vi "Project.vi"(7 "Config in":refnum<class "TAF Proj Config.lvclass">, 8 "error in":errorcluster, 11 "Project":refnum<vi>) -> (0 "error out":errorcluster, 3 "Targets":T1[](array[typedef]))   [LabVIEW 2021, in "TAF Proj Document Type.lvlib" / "Project Parser.lvlib"]
uses:
  <vilib>/Wovalab/AntiDoc/Document Type/Add-ons/LabVIEW TAF Project/Project Parser/Project Parser.lvlib
  <vilib>/Wovalab/AntiDoc/Document Type/Add-ons/LabVIEW TAF Project/TAF Proj Config/TAF Proj Config.lvclass
  <vilib>/Wovalab/AntiDoc/Document Type/Add-ons/LabVIEW TAF Project/Project Parser/Target--cluster.ctl
  <vilib>/Wovalab/AntiDoc/Document Type/Add-ons/LabVIEW TAF Project/Custom Errors/Custom Errors.lvclass
  <vilib>/Wovalab/AntiDoc/Document Type/Add-ons/LabVIEW TAF Project/Classes Overview/Classes Overview.lvclass
  <vilib>/Wovalab/AntiDoc/Document Type/Add-ons/LabVIEW TAF Project/Dqmh Modules Overview/Dqmh Modules Overview.lvclass
  <vilib>/Wovalab/AntiDoc/Document Type/Add-ons/LabVIEW TAF Project/FrontPanelGUI/FrontPanelGUI.lvclass
  <vilib>/Wovalab/AntiDoc/Document Type/Add-ons/LabVIEW TAF Project/Project Parser/Blocs--cluster.ctl
  <vilib>/Wovalab/AntiDoc/Document Type/Add-ons/LabVIEW TAF Project/Dqmh Module/Dqmh Module.lvclass
  <vilib>/Wovalab/AntiDoc/Document Type/Add-ons/LabVIEW TAF Project/Class/Class.lvclass
  <vilib>/Wovalab/AntiDoc/Document Type/Add-ons/LabVIEW TAF Project/Lib/Lib.lvclass
  <vilib>/Wovalab/AntiDoc/Document Type/Add-ons/LabVIEW TAF Project/TAFConfiguration/TAFConfiguration.lvclass
  <vilib>/Wovalab/AntiDoc/Document Type/Add-ons/LabVIEW TAF Project/TAF Proj Config/TAF Proj Config.lvclass/TAF Proj Config.ctl
  <vilib>/Wovalab/AntiDoc/Document Type/Add-ons/LabVIEW TAF Project/TAF Proj Config/Read Scan Dependencies.vi
  <vilib>/Utility/EditLVProj/Edit LVProj.lvlib
  <vilib>/Wovalab/AntiDoc/Progress Bar/Progress Bar.lvlib
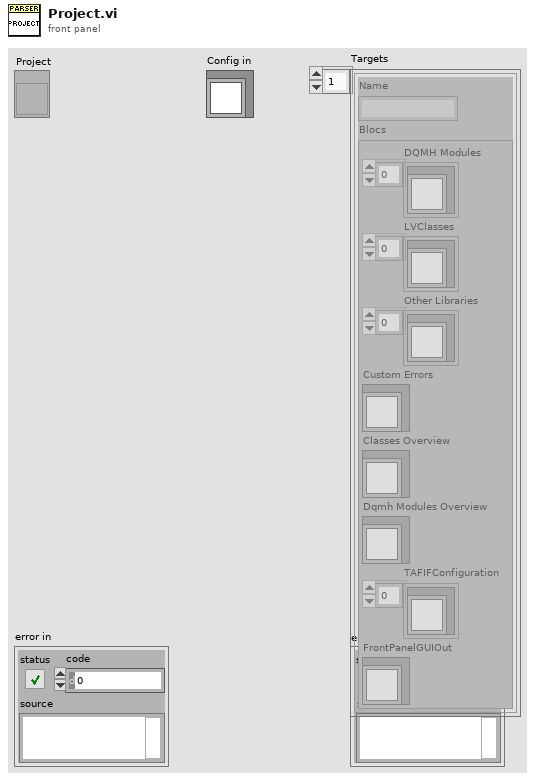
[diagram p1: front panel]
types:
  T1 = typedef "TAF Proj Document Type.lvlib/Project Parser.lvlib/Target--cluster.ctl" = cluster{"Name":string, "Blocs":T2}
  T2 = typedef "TAF Proj Document Type.lvlib/Project Parser.lvlib/Blocs--cluster.ctl" = cluster{"DQMH Modules":refnum<class "Dqmh Module.lvclass">[], "LVClasses":refnum<class "Class.lvclass">[], "Other Libraries":refnum<class "Lib.lvclass">[], "Custom Errors":refnum<class "Custom Errors.lvclass">, "Classes Overview":refnum<class "Classes Overview.lvclass">, "Dqmh Modules Overview":refnum<class "Dqmh Modules Overview.lvclass">, "TAFIFConfiguration":refnum<class "TAFConfiguration.lvclass">[], "FrontPanelGUIOut":refnum<class "FrontPanelGUI.lvclass">}
  T3 = typedef "Edit LVProj.lvlib/Library And VI References.ctl" = cluster{"Target Reference":refnum<vi>, "VI References":refnum<vi>[], "Library References":refnum<vi>[]}
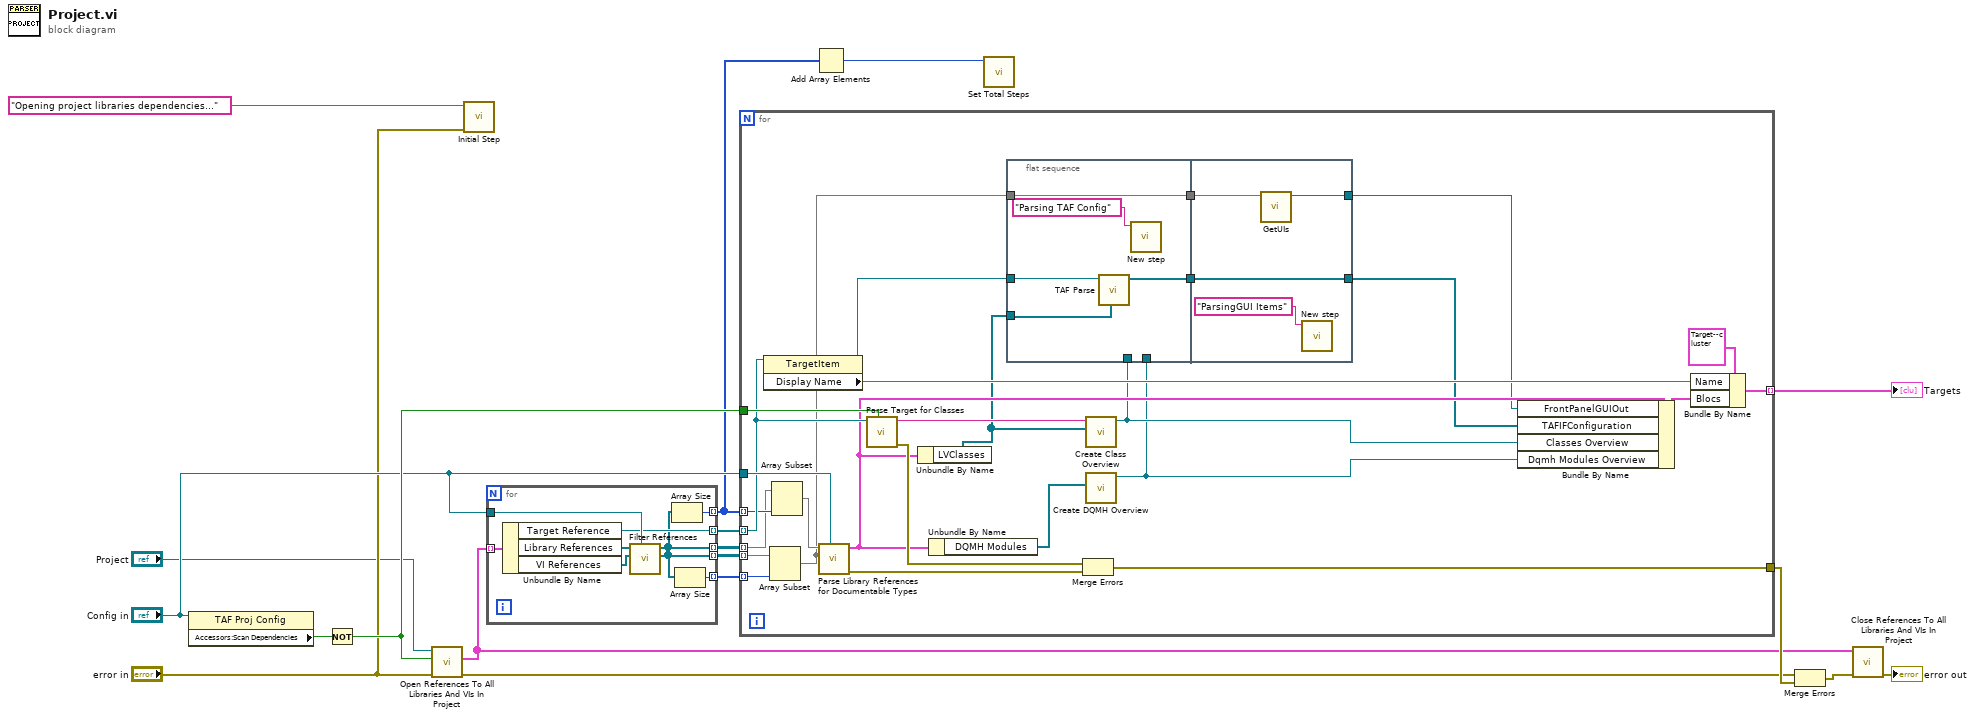
[diagram p0: block diagram]
diagram:
  n1 = property class="TAF Proj Config"(reference="Config in") -> ("Accessors:Scan Dependencies"=w12:bool)  [unwired: 1 in, 2 out]
  n2 = Not(x=w12) -> (.not. x?=w13:bool)
  n3 = call <vilib>:"Open References To All Libraries And VIs In Project.vi"("error in (no error)"="error in", "Exclude Dependencies? (T)"=w13, "Project in"="Project") -> ("error out"=w15:errorcluster, "VI and Library References"=w11:T3[])  [unwired: 6 in, 1 out]
  n4 = call <vilib>:"Initial Step.vi"("error in"="error in", "Description"="Opening project libraries dependencies...") -> ()  [unwired: 9 in, 1 out]
  n5 = for {
    tunnel: w11 -> [w27] mode=indexing
    tunnel: "Config in" -> [w24]
    tunnel: [w23] -> w9 mode=indexing
    tunnel: [w22] -> w8 mode=indexing
    tunnel: [w20] -> w7 mode=indexing
    tunnel: [w21] -> w6 mode=indexing
    tunnel: [w19] -> w5 mode=indexing
    n6 = Unbundle By Name(w27) -> ("Target Reference"=w23:refnum<vi>, "Library References"=w26:refnum<vi>[], "VI References"=w25:refnum<vi>[])
    n7 = call <vilib>:"Filter References.vi"("Config out"=w24, "VI References in"=w25, "Library References in"=w26) -> ("VI References out"=w20:refnum<vi>[], "Library References out"=w22:refnum<vi>[])  [unwired: 7 in]
    n8 = Array Size(array=w22) -> (size(s)=w21:i32)
    n9 = Array Size(array=w20) -> (size(s)=w19:i32)
  }
  n10 = for {
    tunnel: [w53] -> w18
    tunnel: [w50] -> w14 mode=indexing
    tunnel: w13 -> [w47]
    tunnel: "Config in" -> [w46]
    tunnel: w9 -> [w45] mode=indexing
    tunnel: w8 -> [w42] mode=indexing
    tunnel: w7 -> [w40] mode=indexing
    tunnel: w6 -> [w44] mode=indexing
    tunnel: w5 -> [w41] mode=indexing
    n11 = property class="TargetItem"(reference=w45) -> (reference out=w36:refnum<vi>, "Display Name"=w49:string)  [unwired: 1 in, 1 out]
    n12 = Array Subset(array=w40, length=w41) -> (w29:refnum<vi>[])  [unwired: 1 in]
    n13 = Array Subset(array=w42, length=w44) -> (w43:refnum<vi>[])  [unwired: 1 in]
    n14 = call <vilib>:"Parse Library References for Documentable Types.vi"("Config"=w46, "VI References"=w29, "Library References"=w43) -> ("error out"=w54:errorcluster, "Blocs"=w39:T2)  [unwired: 7 in]
    n15 = call <vilib>:"Parse Target for Classes.vi"("exclude dependencies"=w47, "target reference"=w45) -> ("error out"=w52:errorcluster, "Plant UML String"=w37:string)  [unwired: 8 in]
    n16 = Unbundle By Name(w39) -> ("LVClasses"=w34:refnum<class "Class.lvclass">[])
    n17 = Unbundle By Name(w39) -> ("DQMH Modules"=w38:refnum<class "Dqmh Module.lvclass">[])
    n18 = flat-sequence {
      tunnel: w36 -> [w59]
      tunnel: w34 -> [w57]
      tunnel: w33 -> [_]
      tunnel: w32 -> [_]
      tunnel: [w58] -> w31
      tunnel: w29 -> [w56]
      tunnel: [w56] -> w28
      tunnel: [w63] -> w35
      tunnel: w31 -> [w63]
      tunnel: [w62] -> w30
      tunnel: w28 -> [w61]
      frame #0 {
        n19 = call <vilib>:"TAF Parse.vi"("Classes"=w57, "TargetItem in"=w59) -> ("TAFInterfaceConfigurations"=w58:refnum<class "TAFConfiguration.lvclass">[])  [unwired: 9 in]
        n20 = call <vilib>:"New step.vi"("Description"="Parsing TAF Config") -> ()  [unwired: 10 in, 1 out]
      }
      frame #1 {
        n21 = call <vilib>:"GetUIs.vi"("AllVIs"=w61) -> ("TAFProjDocumentType:FrontPanelGUIOut"=w62:refnum<class "FrontPanelGUI.lvclass">)  [unwired: 10 in]
        n22 = call <vilib>:"New step.vi"("Description"="ParsingGUI Items") -> ()  [unwired: 10 in, 1 out]
      }
    }
    n23 = Merge Errors(w52, w54) -> (w53:errorcluster)
    n24 = call <vilib>:"Create Class Overview.vi"("Classes"=w34, "Uml"=w37) -> ("Classes Overview out"=w33:refnum<class "Classes Overview.lvclass">)  [unwired: 8 in, 1 out]
    n25 = call <vilib>:"Create DQMH Overview.vi"("DQMH Modules"=w38) -> ("Dqmh Modules Overview out"=w32:refnum<class "Dqmh Modules Overview.lvclass">)  [unwired: 9 in, 1 out]
    n26 = Bundle By Name(cluster=w39, "FrontPanelGUIOut"=w30, "TAFIFConfiguration"=w35, "Classes Overview"=w33, "Dqmh Modules Overview"=w32) -> (w48:T2)
    n27 = Bundle By Name(cluster=T1 {"Name"="", "Blocs"={"DQMH Modules"=[], "LVClasses"=[], "Other Libraries"=[], "Custom Errors"=refnum, "Classes Overview"=refnum, "Dqmh Modules Overview"=refnum, "TAFIFConfiguration"=[], "FrontPanelGUIOut"=refnum}} ("Target"), "Name"=w49, "Blocs"=w48) -> (w50:T1)
  }
  "Targets" <- w14
  n28 = Add Array Elements(numeric array=w6) -> (sum=w2:i32)
  n29 = call <vilib>:"Set Total Steps.vi"("Total Steps"=w2) -> ()  [unwired: 11 in]
  n30 = Merge Errors(w15, w18) -> (w16:errorcluster)
  n31 = call <vilib>:"Close References To All Libraries And VIs In Project.vi"("error in (no error)"=w16, "VI and Library References"=w11) -> ("error out"=→"error out":errorcluster)  [unwired: 9 in]
